vi "Event Handling Loop.vi"(8 "error in (no error)":errorcluster, 11 "Message Queue":refnum<queue>) -> (0 "dup error in":errorcluster, 3 "dup Message Queue":refnum<queue>)   [LabVIEW 2014]
doc: "Process an error that occurred in the Event Handling Loop, either by ignoring it, or generating an \"Error\" message."
uses:
  Message Queue/Message Cluster.ctl
  Message Queue/Enqueue Message (Single).vi
  Message Queue/Message Queue.lvlib
panel:
  # "LICENSED MATERIALS – PROPERTY OF IBM\nCopyright IBM Corp. 2016,\nALL RIGHTS RESERVED"
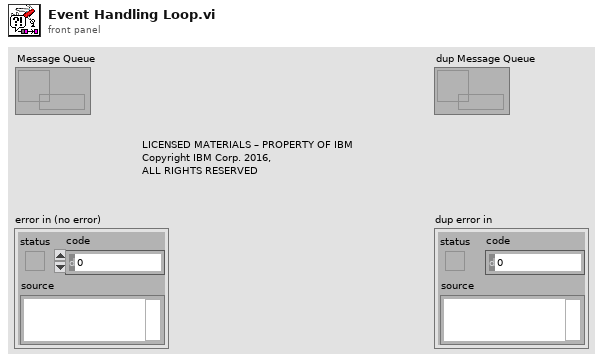
[diagram p1: front panel]
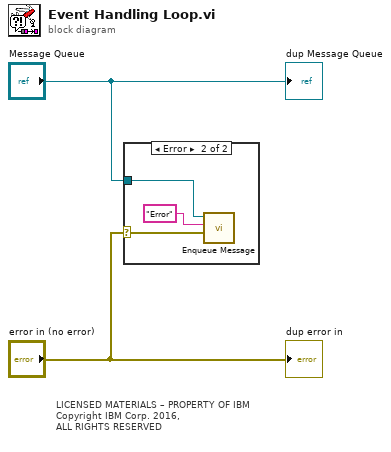
[diagram p0: block diagram]
diagram:
  # "LICENSED MATERIALS – PROPERTY OF IBM\nCopyright IBM Corp. 2016,\nALL RIGHTS RESERVED"
  n1 = case shown="Error" "error in (no error)" {
    selector: "error in (no error)" -> [_ w4]
    tunnel: "Message Queue" -> [_ w3]
    frame No Error {
    }
    frame Error {
      n2 = call-poly "Enqueue Message.vi"("Message Data"=w4, "Message"="Error", "Message Queue"=w3) -> ()  [unwired: 2 in, 7 out]
    }
  }
  "dup Message Queue" <- "Message Queue"
  "dup error in" <- "error in (no error)"
